vi "DisplacementSampleSensorLoop.vi"   [LabVIEW 2016]
uses:
  DisplacementSampleSensorLoopData.ctl
  DisplacementSampleSensorLoopStates.ctl
  DisplacementSample.ctl
  DisplacementErrorSample.ctl
  DisplacementErrorCodes.ctl
  <vilib>/Platform/TimedLoop/XDataNode/timing_clust.ctl
  <vilib>/Platform/TimedLoop/XDataNode/nitl_modes.ctl
  <vilib>/Platform/TimedLoop/XDataNode/wakeup.ctl
  <vilib>/rvi/Emulation/niFpgaSctlEmulationGetInTimedLoop.vi
  <vilib>/rvi/Emulation/niFpgaEmulationReportErrorSimple.vi
  <vilib>/rvi/Emulation/niFpgaGetClockAttributes.vi
  <vilib>/rvi/Emulation/niFpgaCriticalErrorInLSC.vi
  <vilib>/rvi/Emulation/niFpgaEmulationIsFPGAContextNoSignature.vi
  <vilib>/rvi/errors/niFpgaSetErrorForExecOnDevCompSimple.vi
  <vilib>/rvi/eio/common/nirviEmuReportErrorAndStop.vi
  <vilib>/rvi/DataTransferAndStorage/Container/Common/niFpgaContainerGetUniqueNameForEmu.vi
  <vilib>/rvi/FIFO/Fifo_Resource/nirvififoEmulationSetSize.vi
  <vilib>/rvi/FIFO/Fifo_Resource/nirviFifoEmulationQueueMgr.vi
  <instcachedir>/0/nirviFifoEmulationQueueMgr_E5CAEC123FF24DC58D834DCA3CDAA9B5.lvgen/nirviFifoEmulationQueueMgr_E5CAEC123FF24DC58D834DCA3CDAA9B5_004.vi
  <vilib>/Utility/error.llb/Clear Errors.vi
  <vilib>/rvi/FIFO/Fifo_Resource/nirvififoEmulationCreateLock.vi
  <vilib>/rvi/Emulation/niFpgaProcessEmulError.vi
  <vilib>/rvi/FIFO/Fifo_Resource/nirvififoEmulationObtainLock.vi
  <vilib>/rvi/FIFO/Fifo_Resource/nirvififoEmulationReleaseLock.vi
  <vilib>/rvi/occurrence/nirviWaitOnOccurrenceBase.vi
  <vilib>/rvi/errors/nirviReportUnexpectedCaseInternalError.vi
  <vilib>/rvi/errors/nirviReportUnexpectedCaseInternalError (U32).vi
  <vilib>/rvi/FIFO/Fifo_Resource/nirvififoEmulationDetermineInputValidOut.vi
  <instcachedir>/0/nirviFifoEmulationQueueMgr_E5CAEC123FF24DC58D834DCA3CDAA9B5.lvgen/nirviFifoEmulationQueueMgr_E5CAEC123FF24DC58D834DCA3CDAA9B5_009.vi
  <vilib>/rvi/Memory/Memory_Emulation/niFpgaMemoryEmulationCacheClearOnFirstRun.vi
  <vilib>/rvi/Memory/Memory_Emulation/nirvimemoryEmulationManagerCache_MakeExclusive.vi
  <vilib>/rvi/Memory/Memory_Emulation/niFpgaMemoryEmulationValidateCache.vi
  <vilib>/rvi/Memory/Memory_Emulation/nirvimemoryEmulationManagerCache_InsertValue.vi
  <vilib>/rvi/Memory/Memory_Emulation/nirvimemoryEmulationManagerCache_ReleaseExclusive.vi
  <vilib>/rvi/Memory/Memory_Emulation/nirvimemoryEmulationManagerCache_GetValue.vi
  <vilib>/rvi/Memory/Memory_Emulation/nirvimemoryEmulationManagerCache_SetValue.vi
  <vilib>/rvi/eio/common/nirviEmuTemplateMethod_errors.vi
  <instcachedir>/0/nirviFifoEmulationQueueMgr_E5CAEC123FF24DC58D834DCA3CDAA9B5.lvgen/nirviFifoEmulationQueueMgr_E5CAEC123FF24DC58D834DCA3CDAA9B5_028.vi
  <instcachedir>/0/nirviFifoEmulationQueueMgr_E5CAEC123FF24DC58D834DCA3CDAA9B5.lvgen/nirviFifoEmulationQueueMgr_E5CAEC123FF24DC58D834DCA3CDAA9B5_029.vi
  <vilib>/Platform/TimedLoop/XDataNode/XDataNode.xnode
  <vilib>/rvi/DataTransferAndStorage/Container/XNode/niFpgaContainer.xnode
  <vilib>/rvi/FIFO/Fifo_Resource/nirvififoEmulationRead.vi
  <vilib>/rvi/FIFO/Fifo_Resource/nirvififoEmulationWrite.vi
  <vilib>/rvi/DataTransferAndStorage/Register/Emulation/niFpgaRegisterEmulation.vi
  <vilib>/eio/EIONode/EIONode.xnode
  <vilib>/Platform/TimedLoop/XDataNode/XDNodeRunTimeDep.lvlib
types:
  T1 = typedef "DisplacementSampleSensorLoopData.ctl" = cluster{"State":T2, "Sensor":u8, "Negative":bool, "Timestamp":u64, "ErrorNumber":u8, "Timeout":i32, "Sample":T3, "ErrorSample":T4}
  T2 = typedef "DisplacementSampleSensorLoopStates.ctl" = enum16{"WaitForTrigger", "ClearRxFIFO", "WaitForClearComplete", "WriteM", "Write0", "WriteCR", "WriteNL", "ReadFirstCharacter", "ReadDataResponse", "ReadDeliminator", "ReadSign", "ReadHundreds", "ReadTens", "ReadOnes", "ReadDecimal", "ReadTenths", "ReadHundredths", "ReadThousandths", "ReadTenThousandths", "PrepareSample", "MoveSample", "ReadErrorR", "ReadErrorDeliminator1", "ReadErrorM", "ReadError0", "ReadErrorDeliminator2", "ReadErrorNumberTens", "ReadErrorNumberOnes", "ReadErrorCR", "ParseErrorNumber", "ResponseUnknownError", "ResponseInvalidError", "ResponseTimeoutError", "SensorIndicatesInvalidCommandError", "SensorIndicatesCommunicationTimeoutError", "SensorIndicatesDataLengthError", "SensorIndicatesNumberOfParametersError", "SensorIndicatesParameterError", "SensorIndicatesCommunicationError", "SensorIndicatesIDNumberError", "SensorIndicatesExpansionLineError", "SensorIndicatesWriteControlError", "PrepareErrorCode", "MoveErrorCode"}
  T3 = typedef "DisplacementSample.ctl" = cluster{"Timestamp":u64, "TxBytes":u64, "RxBytes":u64, "TxFrames":u64, "RxFrames":u64, "Sensor1Raw":i32, "Sensor2Raw":i32, "Sensor3Raw":i32, "Sensor4Raw":i32, "Sensor5Raw":i32, "Sensor6Raw":i32, "Sensor7Raw":i32, "Sensor8Raw":i32, "Sensor1Eng":sgl, "Sensor2Eng":sgl, "Sensor3Eng":sgl, "Sensor4Eng":sgl, "Sensor5Eng":sgl, "Sensor6Eng":sgl, "Sensor7Eng":sgl, "Sensor8Eng":sgl, "PositionX":sgl, "PositionY":sgl, "PositionZ":sgl, "RotationX":sgl, "RotationY":sgl, "RotationZ":sgl}
  T4 = typedef "DisplacementErrorSample.ctl" = cluster{"Timestamp":u64, "TxBytes":u64, "RxBytes":u64, "TxFrames":u64, "RxFrames":u64, "ErrorCode":T5}
  T5 = typedef "DisplacementErrorCodes.ctl" = enum16{"None", "ResponseUnknownError", "ResponseInvalidError", "ResponseTimeoutError", "SensorIndicatesInvalidCommandError", "SensorIndicatesCommunicationTimeoutError", "SensorIndicatesDataLengthError", "SensorIndicatesNumberOfParametersError", "SensorIndicatesParameterError", "SensorIndicatesCommunicationError", "SensorIndicatesIDNumberError", "SensorIndicatesExpansionLineError", "SensorIndicatesWriteControlError"}
  T6 = typedef "XDNodeRunTimeDep.lvlib/timing_clust.ctl" = cluster{"Expected End [f-1]":u64, "Actual End [f-1]":u64, "Finished Late? [f-1]":bool, "Expected End [i-1]":u64, "Actual End [i-1]":u64, "Finished Late? [i-1]":bool, "Expected Start [i]":u64, "Actual Start [i]":u64, "Expected Start [f]":u64, "Actual Start [f]":u64, "Source Name":string, "Structure Name":string, "Period":i64, "Deadline":i64, "Offset":i64, "Start":i64, "Priority":i32, "Timeout":i32, "Mode":T7, "Wakeup Reason":T8, "Error":errorcluster, "Source Type":string, "Secondary Source Type":string, "Global End Time":u64, "Global Start Time":u64, "Frame Duration":u64, "Iteration Duration":u64, "Assigned CPU":i32, "I/O Scan Engine Mode":u32}
  T7 = typedef "XDNodeRunTimeDep.lvlib/nitl_modes.ctl" = enum32{"No Change", "Process missed periods, maintain original phase", "Discard missed periods, maintain original phase", "Process missed periods, ignore original phase", "Discard missed periods, ignore original phase"}
  T8 = typedef "XDNodeRunTimeDep.lvlib/wakeup.ctl" = enum32{"Normal", "Aborted", "Asynchronous wakeup", "Timing source error", "Timed loop error", "Timeout"}
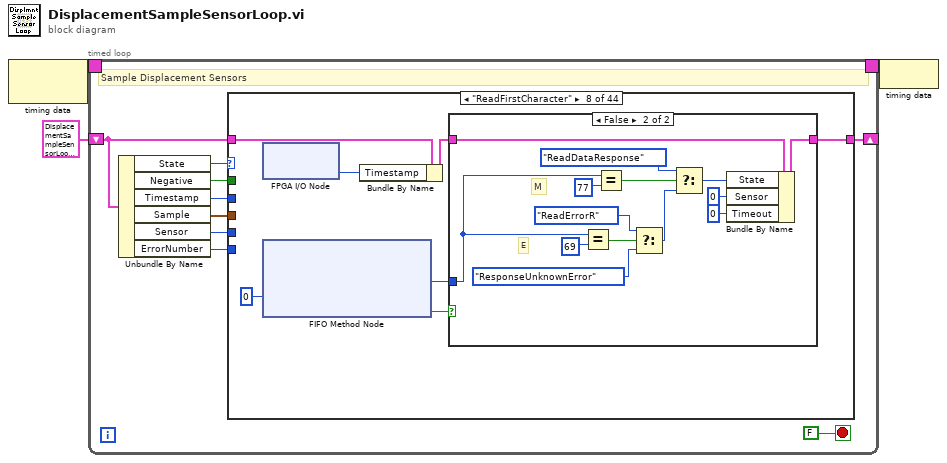
[diagram p0: block diagram]
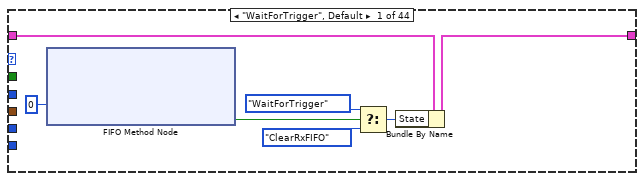
[diagram p2: hidden frame]
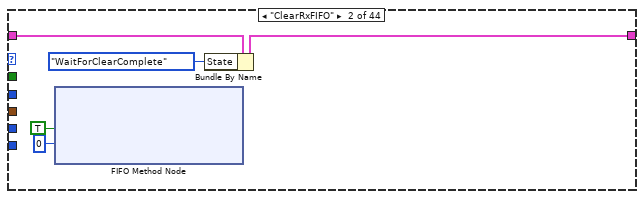
[diagram p3: hidden frame]
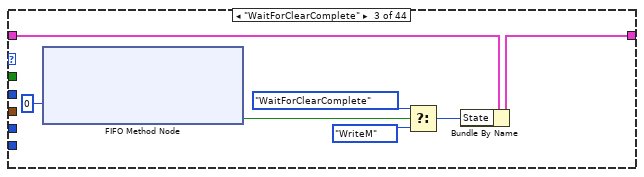
[diagram p4: hidden frame]
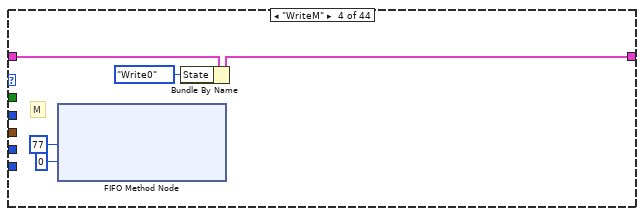
[diagram p5: hidden frame]
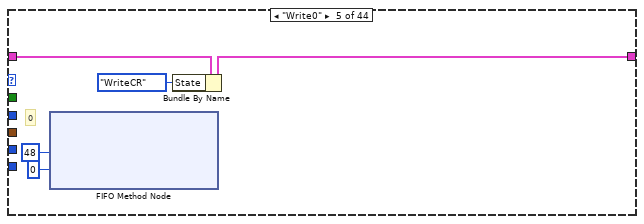
[diagram p6: hidden frame]
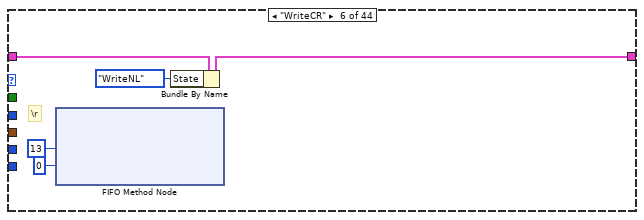
[diagram p7: hidden frame]
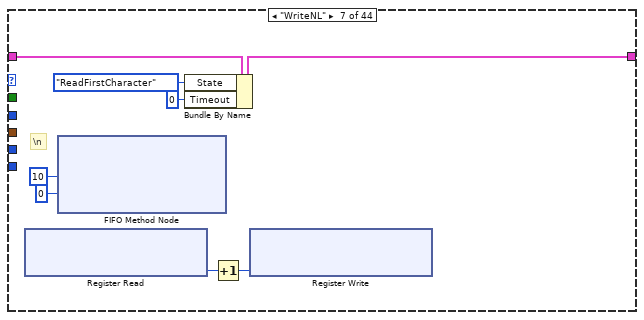
[diagram p8: hidden frame]
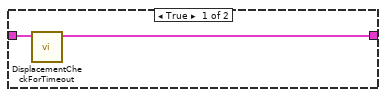
[diagram p9: hidden frame]
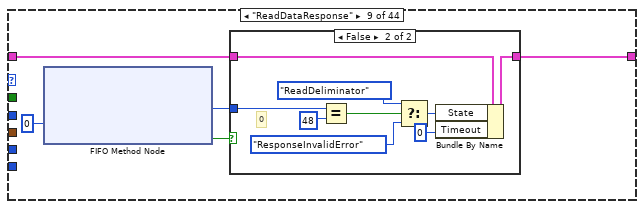
[diagram p10: hidden frame]
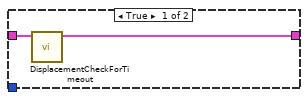
[diagram p11: hidden frame]
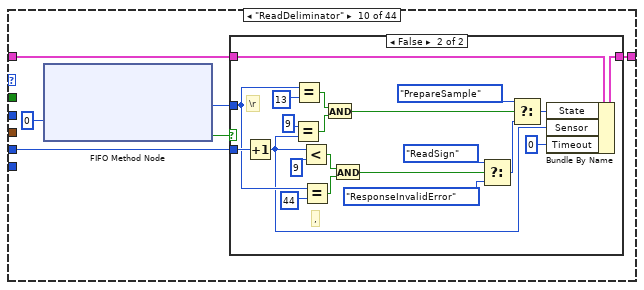
[diagram p12: hidden frame]
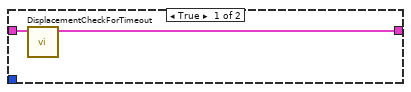
[diagram p13: hidden frame]
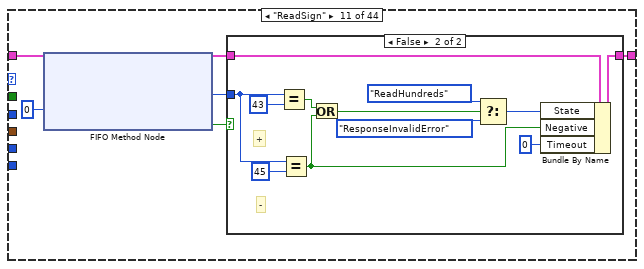
[diagram p14: hidden frame]
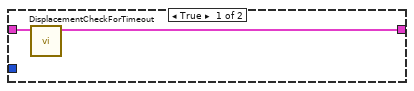
[diagram p15: hidden frame]
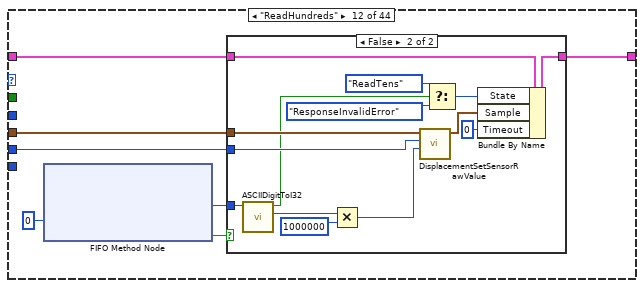
[diagram p16: hidden frame]
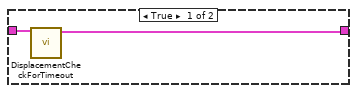
[diagram p17: hidden frame]
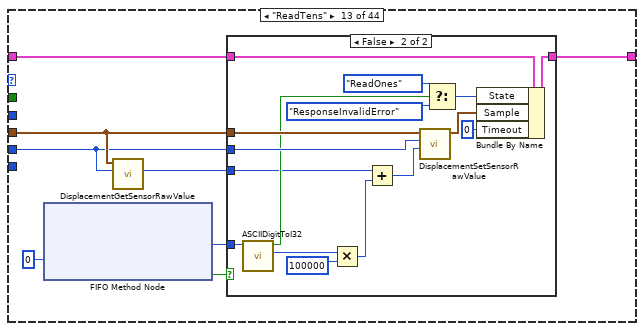
[diagram p18: hidden frame]
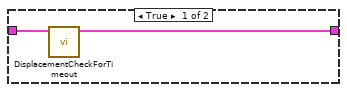
[diagram p19: hidden frame]
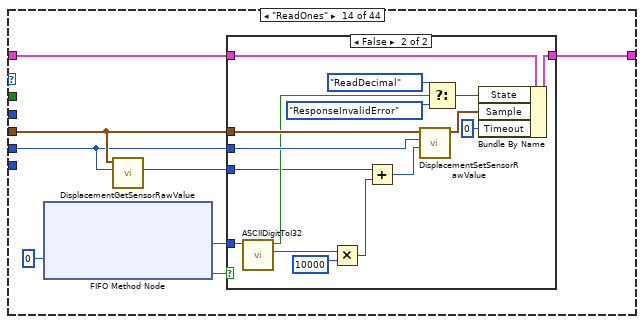
[diagram p20: hidden frame]
diagram:
  n1 = node-c288() -> (w3:T6)  [unwired: 1 in]
  n2 = timed-loop {
    timing: w3 -> [_]
    timing-out: [_] -> w2
    shift-right: [w12] -> _
    shift-left: T1 {"State"=enum."WaitForTrigger", "Sensor"=0, "Negative"=FALSE, "Timestamp"=0, "ErrorNumber"=0, "Timeout"=0, "Sample"={"Timestamp"=0, "TxBytes"=0, "RxBytes"=0, "TxFrames"=0, "RxFrames"=0, "Sensor1Raw"=0, "Sensor2Raw"=0, "Sensor3Raw"=0, "Sensor4Raw"=0, "Sensor5Raw"=0, "Sensor6Raw"=0, "Sensor7Raw"=0, "Sensor8Raw"=0, "Sensor1Eng"=0.0, "Sensor2Eng"=0.0, "Sensor3Eng"=0.0, "Sensor4Eng"=0.0, "Sensor5Eng"=0.0, "Sensor6Eng"=0.0, "Sensor7Eng"=0.0, "Sensor8Eng"=0.0, "PositionX"=0.0, "PositionY"=0.0, "PositionZ"=0.0, "RotationX"=0.0, "RotationY"=0.0, "RotationZ"=0.0}, "ErrorSample"={"Timestamp"=0, "TxBytes"=0, "RxBytes"=0, "TxFrames"=0, "RxFrames"=0, "ErrorCode"=enum."None"}} ("DisplacementData") -> [w11]
    stop <- FALSE stop-if-true
    # "Sample Displacement Sensors"
    n3 = Unbundle By Name(w11) -> ("State"=w10:T2, "Negative"=w9:bool, "Timestamp"=w7:u64, "Sample"=w8:T3, "Sensor"=w6:u8, "ErrorNumber"=w5:u8)
    n4 = case shown="\"ReadFirstCharacter\"" w10 {
      tunnel: [w16 w23 w30 w35 w40 w45 w53 w61 w81 w98 w126 w147 w171 w197 w220 w239 w265 w291 w317 w343 w350 w354 w370 w386 w402 w418 w434 w454 w473 w488 w502 w506 w510 w514 w518 w522 w526 w530 w534 w538 w542 w546 w556 w563] -> w12
      tunnel: w11 -> [w19 w24 w31 w36 w41 w46 w54 w57 w82 w99 w127 w148 w172 w198 w221 w240 w266 w292 w318 w344 w347 w355 w371 w387 w403 w419 w435 w455 w474 w489 w503 w507 w511 w515 w519 w523 w527 w531 w535 w539 w543 w547 w557 w560]
      tunnel: w9 -> [_ _ _ _ _ _ _ _ _ _ _ _ _ _ _ _ _ _ _ _ _ _ _ _ _ _ _ _ _ _ _ _ _ _ _ _ _ _ _ _ _ _ _ _]
      tunnel: w8 -> [_ _ _ _ _ _ _ _ _ _ _ w143 w167 w193 _ w235 w261 w287 w313 _ _ _ _ _ _ _ _ _ _ _ _ _ _ _ _ _ _ _ _ _ _ _ _ _]
      tunnel: w7 -> [_ _ _ _ _ _ _ _ _ _ _ _ _ _ _ _ _ _ _ w335 _ _ _ _ _ _ _ _ _ _ _ _ _ _ _ _ _ _ _ _ _ _ w548 _]
      tunnel: w6 -> [_ _ _ _ _ _ _ _ _ w94 _ w142 w166 w192 _ w234 w260 w286 w312 _ _ _ _ _ _ _ _ _ _ _ _ _ _ _ _ _ _ _ _ _ _ _ _ _]
      tunnel: w5 -> [_ _ _ _ _ _ _ _ _ _ _ _ _ _ _ _ _ _ _ _ _ _ _ _ _ _ _ w450 _ w486 _ _ _ _ _ _ _ _ _ _ _ _ _ _]
      frame "WaitForTrigger", Default {
        n5 = xnode ("FIFO Method Node")("Timeout"=0) -> ("Timed Out?"=w14:bool)  [unwired: 1 in, 2 out]
        n6 = Select(t=DisplacementSampleSensorLoopStates."WaitForTrigger" ("DisplacementStates"), s=w14, f=DisplacementSampleSensorLoopStates."ClearRxFIFO") -> (s? t:f=w17:T2)
        n7 = Bundle By Name(cluster=w19, "State"=w17) -> (w16:T1)
      }
      frame "ClearRxFIFO" {
        n8 = xnode ("FIFO Method Node")("Element"=TRUE, "Timeout"=0) -> ()  [unwired: 1 in, 2 out]
        n9 = Bundle By Name(cluster=w24, "State"=DisplacementSampleSensorLoopStates."WaitForClearComplete") -> (w23:T1)
      }
      frame "WaitForClearComplete" {
        n10 = xnode ("FIFO Method Node")("Timeout"=0) -> ("Timed Out?"=w26:bool)  [unwired: 1 in, 2 out]
        n11 = Select(t=DisplacementSampleSensorLoopStates."WaitForClearComplete" ("State"), s=w26, f=DisplacementSampleSensorLoopStates."WriteM") -> (s? t:f=w28:T2)
        n12 = Bundle By Name(cluster=w31, "State"=w28) -> (w30:T1)
      }
      frame "WriteM" {
        # "M"
        n13 = xnode ("FIFO Method Node")("Element"=u8 77, "Timeout"=0) -> ()  [unwired: 1 in, 2 out]
        n14 = Bundle By Name(cluster=w36, "State"=DisplacementSampleSensorLoopStates."Write0" ("f")) -> (w35:T1)
      }
      frame "Write0" {
        # "0"
        n15 = xnode ("FIFO Method Node")("Element"=u8 48, "Timeout"=0) -> ()  [unwired: 1 in, 2 out]
        n16 = Bundle By Name(cluster=w41, "State"=DisplacementSampleSensorLoopStates."WriteCR" ("f")) -> (w40:T1)
      }
      frame "WriteCR" {
        # "\\r"
        n17 = xnode ("FIFO Method Node")("Element"=u8 13, "Timeout"=0) -> ()  [unwired: 1 in, 2 out]
        n18 = Bundle By Name(cluster=w46, "State"=DisplacementSampleSensorLoopStates."WriteNL" ("f")) -> (w45:T1)
      }
      frame "WriteNL" {
        # "\\n"
        n19 = xnode ("Register Read")() -> ("Data"=w48:u64)  [unwired: 1 in, 1 out]
        n20 = xnode ("FIFO Method Node")("Element"=u8 10, "Timeout"=0) -> ()  [unwired: 1 in, 2 out]
        n21 = Bundle By Name(cluster=w54, "State"=DisplacementSampleSensorLoopStates."ReadFirstCharacter", "Timeout"=0) -> (w53:T1)
        n22 = Increment(x=w48) -> (x+1=w49:u64)
        n23 = xnode ("Register Write")("Data"=w49) -> ()  [unwired: 1 in, 1 out]
      }
      frame "ReadFirstCharacter" {
        n24 = xnode "FPGA I/O Node"() -> ("Time"=w55:u64)  [unwired: 1 in, 1 out]
        n25 = xnode ("FIFO Method Node")("Timeout"=0) -> ("Element"=w58:u8, "Timed Out?"=w59:bool)  [unwired: 1 in, 1 out]
        n26 = Bundle By Name(cluster=w57, "Timestamp"=w55) -> (w56:T1)
        n27 = case shown="False" w59 {
          tunnel: w56 -> [w63 w64]
          tunnel: [w62 w77] -> w61
          tunnel: w58 -> [_ w70]
          frame True {
            n28 = call "DisplacementCheckForTimeout.vi"("DisplacementSampleSensorLoopData in"=w63) -> ("DisplacementSampleSensorLoopData out"=w62:T1)  [unwired: 10 in]
          }
          frame False {
            # "E"
            # "M"
            n29 = Equal?(x=w70, y=u8 69) -> (x = y?=w71:bool)
            n30 = Equal?(x=w70, y=u8 77) -> (x = y?=w75:bool)
            n31 = Select(t=DisplacementSampleSensorLoopStates."ReadErrorR", s=w71, f=DisplacementSampleSensorLoopStates."ResponseUnknownError") -> (s? t:f=w68:T2)
            n32 = Select(t=DisplacementSampleSensorLoopStates."ReadDataResponse" ("State"), s=w75, f=w68) -> (s? t:f=w74:T2)
            n33 = Bundle By Name(cluster=w64, "State"=w74, "Sensor"=u8 0, "Timeout"=0) -> (w77:T1)
          }
        }
      }
      frame "ReadDataResponse" {
        n34 = xnode ("FIFO Method Node")("Timeout"=0) -> ("Element"=w78:u8, "Timed Out?"=w79:bool)  [unwired: 1 in, 1 out]
        n35 = case shown="False" w79 {
          tunnel: w82 -> [w84 w93]
          tunnel: [w83 w92] -> w81
          tunnel: w78 -> [_ w87]
          frame True {
            n36 = call "DisplacementCheckForTimeout.vi"("DisplacementSampleSensorLoopData in"=w84) -> ("DisplacementSampleSensorLoopData out"=w83:T1)  [unwired: 10 in]
          }
          frame False {
            # "0"
            n37 = Equal?(x=w87, y=u8 48) -> (x = y?=w90:bool)
            n38 = Select(t=DisplacementSampleSensorLoopStates."ReadDeliminator" ("State"), s=w90, f=DisplacementSampleSensorLoopStates."ResponseInvalidError") -> (s? t:f=w89:T2)
            n39 = Bundle By Name(cluster=w93, "State"=w89, "Timeout"=0) -> (w92:T1)
          }
        }
      }
      frame "ReadDeliminator" {
        n40 = xnode ("FIFO Method Node")("Timeout"=0) -> ("Element"=w95:u8, "Timed Out?"=w96:bool)  [unwired: 1 in, 1 out]
        n41 = case shown="False" w96 {
          tunnel: w99 -> [w101 w122]
          tunnel: [w100 w121] -> w98
          tunnel: w95 -> [_ w111]
          tunnel: w94 -> [_ w118]
          frame True {
            n42 = call "DisplacementCheckForTimeout.vi"("DisplacementSampleSensorLoopData in"=w101) -> ("DisplacementSampleSensorLoopData out"=w100:T1)  [unwired: 10 in]
          }
          frame False {
            # "\\r"
            # ","
            n43 = Increment(x=w118) -> (x+1=w103:u8)
            n44 = Equal?(x=u8 9, y=w103) -> (x = y?=w110:bool)
            n45 = Equal?(x=w111, y=u8 13) -> (x = y?=w109:bool)
            n46 = Less?(x=w103, y=u8 9) -> (x < y?=w116:bool)
            n47 = Equal?(x=w111, y=u8 44) -> (x = y?=w115:bool)
            n48 = And(x=w109, y=w110) -> (x .and. y?=w107:bool)
            n49 = And(x=w116, y=w115) -> (x .and. y?=w104:bool)
            n50 = Select(t=DisplacementSampleSensorLoopStates."ReadSign" ("State"), s=w104, f=DisplacementSampleSensorLoopStates."ResponseInvalidError") -> (s? t:f=w108:T2)
            n51 = Select(t=DisplacementSampleSensorLoopStates."PrepareSample", s=w107, f=w108) -> (s? t:f=w105:T2)
            n52 = Bundle By Name(cluster=w122, "State"=w105, "Sensor"=w103, "Timeout"=0) -> (w121:T1)
          }
        }
      }
      frame "ReadSign" {
        n53 = xnode ("FIFO Method Node")("Timeout"=0) -> ("Element"=w123:u8, "Timed Out?"=w124:bool)  [unwired: 1 in, 1 out]
        n54 = case shown="False" w124 {
          tunnel: w127 -> [w129 w141]
          tunnel: [w128 w140] -> w126
          tunnel: w123 -> [_ w137]
          frame True {
            n55 = call "DisplacementCheckForTimeout.vi"("DisplacementSampleSensorLoopData in"=w129) -> ("DisplacementSampleSensorLoopData out"=w128:T1)  [unwired: 10 in]
          }
          frame False {
            # "+"
            # "-"
            n56 = Equal?(x=w137, y=u8 43) -> (x = y?=w138:bool)
            n57 = Equal?(x=w137, y=u8 45) -> (x = y?=w135:bool)
            n58 = Or(x=w138, y=w135) -> (x .or. y?=w134:bool)
            n59 = Select(t=DisplacementSampleSensorLoopStates."ReadHundreds" ("State"), s=w134, f=DisplacementSampleSensorLoopStates."ResponseInvalidError") -> (s? t:f=w132:T2)
            n60 = Bundle By Name(cluster=w141, "State"=w132, "Negative"=w135, "Timeout"=0) -> (w140:T1)
          }
        }
      }
      frame "ReadHundreds" {
        n61 = xnode ("FIFO Method Node")("Timeout"=0) -> ("Element"=w144:u8, "Timed Out?"=w145:bool)  [unwired: 1 in, 1 out]
        n62 = case shown="False" w145 {
          tunnel: w148 -> [w150 w164]
          tunnel: [w149 w163] -> w147
          tunnel: w144 -> [_ w154]
          tunnel: w143 -> [_ w157]
          tunnel: w142 -> [_ w155]
          frame True {
            n63 = call "DisplacementCheckForTimeout.vi"("DisplacementSampleSensorLoopData in"=w150) -> ("DisplacementSampleSensorLoopData out"=w149:T1)  [unwired: 10 in]
          }
          frame False {
            n64 = call "ASCIIDigitToI32.vi"("Value"=w154) -> ("Number"=w152:i32, "Valid"=w153:bool)  [unwired: 9 in]
            n65 = Multiply(x=w152, y=1000000) -> (x*y=w158:i32)
            n66 = call "DisplacementSetSensorRawValue.vi"("Value"=w158, "Sensor"=w155, "DisplacementSample in"=w157) -> ("DisplacementSample out"=w156:T3)  [unwired: 8 in]
            n67 = Select(t=DisplacementSampleSensorLoopStates."ReadTens" ("State"), s=w153, f=DisplacementSampleSensorLoopStates."ResponseInvalidError" ("State")) -> (s? t:f=w161:T2)
            n68 = Bundle By Name(cluster=w164, "State"=w161, "Sample"=w156, "Timeout"=0) -> (w163:T1)
          }
        }
      }
      frame "ReadTens" {
        n69 = xnode ("FIFO Method Node")("Timeout"=0) -> ("Element"=w168:u8, "Timed Out?"=w169:bool)  [unwired: 1 in, 1 out]
        n70 = call "DisplacementGetSensorRawValue.vi"("Sensor"=w166, "DisplacementSample"=w167) -> ("Value"=w165:i32)  [unwired: 9 in]
        n71 = case shown="False" w169 {
          tunnel: w172 -> [w174 w190]
          tunnel: [w173 w189] -> w171
          tunnel: w168 -> [_ w181]
          tunnel: w167 -> [_ w184]
          tunnel: w166 -> [_ w182]
          tunnel: w165 -> [_ w178]
          frame True {
            n72 = call "DisplacementCheckForTimeout.vi"("DisplacementSampleSensorLoopData in"=w174) -> ("DisplacementSampleSensorLoopData out"=w173:T1)  [unwired: 10 in]
          }
          frame False {
            n73 = call "ASCIIDigitToI32.vi"("Value"=w181) -> ("Number"=w179:i32, "Valid"=w180:bool)  [unwired: 9 in]
            n74 = Multiply(x=w179, y=100000) -> (x*y=w176:i32)
            n75 = Add(x=w178, y=w176) -> (x+y=w177:i32)
            n76 = call "DisplacementSetSensorRawValue.vi"("Value"=w177, "Sensor"=w182, "DisplacementSample in"=w184) -> ("DisplacementSample out"=w183:T3)  [unwired: 8 in]
            n77 = Select(t=DisplacementSampleSensorLoopStates."ReadOnes" ("State"), s=w180, f=DisplacementSampleSensorLoopStates."ResponseInvalidError" ("State")) -> (s? t:f=w187:T2)
            n78 = Bundle By Name(cluster=w190, "State"=w187, "Sample"=w183, "Timeout"=0) -> (w189:T1)
          }
        }
      }
      frame "ReadOnes" {
        n79 = xnode ("FIFO Method Node")("Timeout"=0) -> ("Element"=w194:u8, "Timed Out?"=w195:bool)  [unwired: 1 in, 1 out]
        n80 = call "DisplacementGetSensorRawValue.vi"("Sensor"=w192, "DisplacementSample"=w193) -> ("Value"=w191:i32)  [unwired: 9 in]
        n81 = case shown="False" w195 {
          tunnel: w198 -> [w200 w216]
          tunnel: [w199 w215] -> w197
          tunnel: w194 -> [_ w207]
          tunnel: w193 -> [_ w210]
          tunnel: w192 -> [_ w208]
          tunnel: w191 -> [_ w204]
          frame True {
            n82 = call "DisplacementCheckForTimeout.vi"("DisplacementSampleSensorLoopData in"=w200) -> ("DisplacementSampleSensorLoopData out"=w199:T1)  [unwired: 10 in]
          }
          frame False {
            n83 = call "ASCIIDigitToI32.vi"("Value"=w207) -> ("Number"=w205:i32, "Valid"=w206:bool)  [unwired: 9 in]
            n84 = Multiply(x=w205, y=10000) -> (x*y=w202:i32)
            n85 = Add(x=w204, y=w202) -> (x+y=w203:i32)
            n86 = call "DisplacementSetSensorRawValue.vi"("Value"=w203, "Sensor"=w208, "DisplacementSample in"=w210) -> ("DisplacementSample out"=w209:T3)  [unwired: 8 in]
            n87 = Select(t=DisplacementSampleSensorLoopStates."ReadDecimal" ("State"), s=w206, f=DisplacementSampleSensorLoopStates."ResponseInvalidError" ("State")) -> (s? t:f=w213:T2)
            n88 = Bundle By Name(cluster=w216, "State"=w213, "Sample"=w209, "Timeout"=0) -> (w215:T1)
          }
        }
      }
      frame "ReadDecimal" {
        n89 = xnode ("FIFO Method Node")("Timeout"=0) -> ("Element"=w217:u8, "Timed Out?"=w218:bool)  [unwired: 1 in, 1 out]
        n90 = case shown="False" w218 {
          tunnel: w221 -> [w223 w232]
          tunnel: [w222 w231] -> w220
          tunnel: w217 -> [_ w227]
          frame True {
            n91 = call "DisplacementCheckForTimeout.vi"("DisplacementSampleSensorLoopData in"=w223) -> ("DisplacementSampleSensorLoopData out"=w222:T1)  [unwired: 10 in]
          }
          frame False {
            # "."
            n92 = Equal?(x=w227, y=u8 46) -> (x = y?=w225:bool)
            n93 = Select(t=DisplacementSampleSensorLoopStates."ReadTenths" ("State"), s=w225, f=DisplacementSampleSensorLoopStates."ResponseInvalidError" ("State")) -> (s? t:f=w230:T2)
            n94 = Bundle By Name(cluster=w232, "State"=w230, "Timeout"=0) -> (w231:T1)
          }
        }
      }
      frame "ReadTenths" {
        n95 = xnode ("FIFO Method Node")("Timeout"=0) -> ("Element"=w236:u8, "Timed Out?"=w237:bool)  [unwired: 1 in, 1 out]
        n96 = call "DisplacementGetSensorRawValue.vi"("Sensor"=w234, "DisplacementSample"=w235) -> ("Value"=w233:i32)  [unwired: 9 in]
        n97 = case shown="False" w237 {
          tunnel: w240 -> [w242 w258]
          tunnel: [w241 w257] -> w239
          tunnel: w236 -> [_ w249]
          tunnel: w235 -> [_ w252]
          tunnel: w234 -> [_ w250]
          tunnel: w233 -> [_ w246]
          frame True {
            n98 = call "DisplacementCheckForTimeout.vi"("DisplacementSampleSensorLoopData in"=w242) -> ("DisplacementSampleSensorLoopData out"=w241:T1)  [unwired: 10 in]
          }
          frame False {
            n99 = call "ASCIIDigitToI32.vi"("Value"=w249) -> ("Number"=w247:i32, "Valid"=w248:bool)  [unwired: 9 in]
            n100 = Multiply(x=w247, y=1000) -> (x*y=w244:i32)
            n101 = Add(x=w246, y=w244) -> (x+y=w245:i32)
            n102 = call "DisplacementSetSensorRawValue.vi"("Value"=w245, "Sensor"=w250, "DisplacementSample in"=w252) -> ("DisplacementSample out"=w251:T3)  [unwired: 8 in]
            n103 = Select(t=DisplacementSampleSensorLoopStates."ReadHundredths" ("State"), s=w248, f=DisplacementSampleSensorLoopStates."ResponseInvalidError" ("State")) -> (s? t:f=w255:T2)
            n104 = Bundle By Name(cluster=w258, "State"=w255, "Sample"=w251, "Timeout"=0) -> (w257:T1)
          }
        }
      }
      frame "ReadHundredths" {
        n105 = xnode ("FIFO Method Node")("Timeout"=0) -> ("Element"=w262:u8, "Timed Out?"=w263:bool)  [unwired: 1 in, 1 out]
        n106 = call "DisplacementGetSensorRawValue.vi"("Sensor"=w260, "DisplacementSample"=w261) -> ("Value"=w259:i32)  [unwired: 9 in]
        n107 = case shown="False" w263 {
          tunnel: w266 -> [w268 w284]
          tunnel: [w267 w283] -> w265
          tunnel: w262 -> [_ w275]
          tunnel: w261 -> [_ w278]
          tunnel: w260 -> [_ w276]
          tunnel: w259 -> [_ w272]
          frame True {
            n108 = call "DisplacementCheckForTimeout.vi"("DisplacementSampleSensorLoopData in"=w268) -> ("DisplacementSampleSensorLoopData out"=w267:T1)  [unwired: 10 in]
          }
          frame False {
            n109 = call "ASCIIDigitToI32.vi"("Value"=w275) -> ("Number"=w273:i32, "Valid"=w274:bool)  [unwired: 9 in]
            n110 = Multiply(x=w273, y=100) -> (x*y=w270:i32)
            n111 = Add(x=w272, y=w270) -> (x+y=w271:i32)
            n112 = call "DisplacementSetSensorRawValue.vi"("Value"=w271, "Sensor"=w276, "DisplacementSample in"=w278) -> ("DisplacementSample out"=w277:T3)  [unwired: 8 in]
            n113 = Select(t=DisplacementSampleSensorLoopStates."ReadThousandths" ("State"), s=w274, f=DisplacementSampleSensorLoopStates."ResponseInvalidError" ("State")) -> (s? t:f=w281:T2)
            n114 = Bundle By Name(cluster=w284, "State"=w281, "Sample"=w277, "Timeout"=0) -> (w283:T1)
          }
        }
      }
      frame "ReadThousandths" {
        n115 = xnode ("FIFO Method Node")("Timeout"=0) -> ("Element"=w288:u8, "Timed Out?"=w289:bool)  [unwired: 1 in, 1 out]
        n116 = call "DisplacementGetSensorRawValue.vi"("Sensor"=w286, "DisplacementSample"=w287) -> ("Value"=w285:i32)  [unwired: 9 in]
        n117 = case shown="False" w289 {
          tunnel: w292 -> [w294 w310]
          tunnel: [w293 w309] -> w291
          tunnel: w288 -> [_ w301]
          tunnel: w287 -> [_ w304]
          tunnel: w286 -> [_ w302]
          tunnel: w285 -> [_ w298]
          frame True {
            n118 = call "DisplacementCheckForTimeout.vi"("DisplacementSampleSensorLoopData in"=w294) -> ("DisplacementSampleSensorLoopData out"=w293:T1)  [unwired: 10 in]
          }
          frame False {
            n119 = call "ASCIIDigitToI32.vi"("Value"=w301) -> ("Number"=w299:i32, "Valid"=w300:bool)  [unwired: 9 in]
            n120 = Multiply(x=w299, y=10) -> (x*y=w296:i32)
            n121 = Add(x=w298, y=w296) -> (x+y=w297:i32)
            n122 = call "DisplacementSetSensorRawValue.vi"("Value"=w297, "Sensor"=w302, "DisplacementSample in"=w304) -> ("DisplacementSample out"=w303:T3)  [unwired: 8 in]
            n123 = Select(t=DisplacementSampleSensorLoopStates."ReadTenThousandths" ("State"), s=w300, f=DisplacementSampleSensorLoopStates."ResponseInvalidError" ("State")) -> (s? t:f=w307:T2)
            n124 = Bundle By Name(cluster=w310, "State"=w307, "Sample"=w303, "Timeout"=0) -> (w309:T1)
          }
        }
      }
      frame "ReadTenThousandths" {
        n125 = xnode ("FIFO Method Node")("Timeout"=0) -> ("Element"=w314:u8, "Timed Out?"=w315:bool)  [unwired: 1 in, 1 out]
        n126 = call "DisplacementGetSensorRawValue.vi"("Sensor"=w312, "DisplacementSample"=w313) -> ("Value"=w311:i32)  [unwired: 9 in]
        n127 = case shown="False" w315 {
          tunnel: w318 -> [w320 w334]
          tunnel: [w319 w333] -> w317
          tunnel: w314 -> [_ w326]
          tunnel: w313 -> [_ w329]
          tunnel: w312 -> [_ w327]
          tunnel: w311 -> [_ w324]
          frame True {
            n128 = call "DisplacementCheckForTimeout.vi"("DisplacementSampleSensorLoopData in"=w320) -> ("DisplacementSampleSensorLoopData out"=w319:T1)  [unwired: 10 in]
          }
          frame False {
            n129 = call "ASCIIDigitToI32.vi"("Value"=w326) -> ("Number"=w322:i32, "Valid"=w325:bool)  [unwired: 9 in]
            n130 = Add(x=w324, y=w322) -> (x+y=w323:i32)
            n131 = call "DisplacementSetSensorRawValue.vi"("Value"=w323, "Sensor"=w327, "DisplacementSample in"=w329) -> ("DisplacementSample out"=w328:T3)  [unwired: 8 in]
            n132 = Select(t=DisplacementSampleSensorLoopStates."ReadDeliminator" ("State"), s=w325, f=DisplacementSampleSensorLoopStates."ResponseInvalidError" ("State")) -> (s? t:f=w332:T2)
            n133 = Bundle By Name(cluster=w334, "State"=w332, "Sample"=w328, "Timeout"=0) -> (w333:T1)
          }
        }
      }
      frame "PrepareSample" {
        n134 = xnode ("Register Read")() -> ("Data"=w341:u64)  [unwired: 1 in, 1 out]
        n135 = xnode ("Register Read")() -> ("Data"=w337:u64)  [unwired: 1 in, 1 out]
        n136 = xnode ("Register Read")() -> ("Data"=w338:u64)  [unwired: 1 in, 1 out]
        n137 = xnode ("Register Read")() -> ("Data"=w336:u64)  [unwired: 1 in, 1 out]
        n138 = Increment(x=w341) -> (x+1=w339:u64)
        n139 = xnode ("Register Write")("Data"=w339) -> ()  [unwired: 1 in, 1 out]
        n140 = Bundle By Name(cluster=w344, "State"=DisplacementSampleSensorLoopStates."MoveSample", "Sensor"=u8 1, "Sample.RxFrames"=w339, "Sample.TxBytes"=w338, "Sample.RxBytes"=w337, "Sample.TxFrames"=w336, "Sample.Timestamp"=w335) -> (w343:T1)
      }
      frame "MoveSample" {
        n141 = Unbundle By Name(w347) -> ("Sample"=w345:T3)
        n142 = xnode ("FIFO Method Node")("Element"=w345, "Timeout"=0) -> ()  [unwired: 1 in, 2 out]
        n143 = Bundle By Name(cluster=w347, "State"=DisplacementSampleSensorLoopStates."WaitForTrigger", "Sensor"=u8 1) -> (w350:T1)
      }
      frame "ReadErrorR" {
        n144 = xnode ("FIFO Method Node")("Timeout"=0) -> ("Element"=w351:u8, "Timed Out?"=w352:bool)  [unwired: 1 in, 1 out]
        n145 = case shown="False" w352 {
          tunnel: w355 -> [w357 w366]
          tunnel: [w356 w365] -> w354
          tunnel: w351 -> [_ w360]
          frame True {
            n146 = call "DisplacementCheckForTimeout.vi"("DisplacementSampleSensorLoopData in"=w357) -> ("DisplacementSampleSensorLoopData out"=w356:T1)  [unwired: 10 in]
          }
          frame False {
            # "R"
            n147 = Equal?(x=w360, y=u8 82) -> (x = y?=w363:bool)
            n148 = Select(t=DisplacementSampleSensorLoopStates."ReadErrorDeliminator1" ("State"), s=w363, f=DisplacementSampleSensorLoopStates."ResponseInvalidError") -> (s? t:f=w362:T2)
            n149 = Bundle By Name(cluster=w366, "State"=w362, "Timeout"=0) -> (w365:T1)
          }
        }
      }
      frame "ReadErrorDeliminator1" {
        n150 = xnode ("FIFO Method Node")("Timeout"=0) -> ("Element"=w367:u8, "Timed Out?"=w368:bool)  [unwired: 1 in, 1 out]
        n151 = case shown="False" w368 {
          tunnel: w371 -> [w373 w382]
          tunnel: [w372 w381] -> w370
          tunnel: w367 -> [_ w377]
          frame True {
            n152 = call "DisplacementCheckForTimeout.vi"("DisplacementSampleSensorLoopData in"=w373) -> ("DisplacementSampleSensorLoopData out"=w372:T1)  [unwired: 10 in]
          }
          frame False {
            # ","
            n153 = Equal?(x=w377, y=u8 44) -> (x = y?=w376:bool)
            n154 = Select(t=DisplacementSampleSensorLoopStates."ReadErrorM" ("State"), s=w376, f=DisplacementSampleSensorLoopStates."ResponseInvalidError") -> (s? t:f=w375:T2)
            n155 = Bundle By Name(cluster=w382, "State"=w375, "Timeout"=0) -> (w381:T1)
          }
        }
      }
      frame "ReadErrorM" {
        n156 = xnode ("FIFO Method Node")("Timeout"=0) -> ("Element"=w383:u8, "Timed Out?"=w384:bool)  [unwired: 1 in, 1 out]
        n157 = case shown="False" w384 {
          tunnel: w387 -> [w389 w398]
          tunnel: [w388 w397] -> w386
          tunnel: w383 -> [_ w392]
          frame True {
            n158 = call "DisplacementCheckForTimeout.vi"("DisplacementSampleSensorLoopData in"=w389) -> ("DisplacementSampleSensorLoopData out"=w388:T1)  [unwired: 10 in]
          }
          frame False {
            # "M"
            n159 = Equal?(x=w392, y=u8 77) -> (x = y?=w395:bool)
            n160 = Select(t=DisplacementSampleSensorLoopStates."ReadError0" ("State"), s=w395, f=DisplacementSampleSensorLoopStates."ResponseInvalidError") -> (s? t:f=w394:T2)
            n161 = Bundle By Name(cluster=w398, "State"=w394, "Timeout"=0) -> (w397:T1)
          }
        }
      }
      frame "ReadError0" {
        n162 = xnode ("FIFO Method Node")("Timeout"=0) -> ("Element"=w399:u8, "Timed Out?"=w400:bool)  [unwired: 1 in, 1 out]
        n163 = case shown="False" w400 {
          tunnel: w403 -> [w405 w414]
          tunnel: [w404 w413] -> w402
          tunnel: w399 -> [_ w408]
          frame True {
            n164 = call "DisplacementCheckForTimeout.vi"("DisplacementSampleSensorLoopData in"=w405) -> ("DisplacementSampleSensorLoopData out"=w404:T1)  [unwired: 10 in]
          }
          frame False {
            # "0"
            n165 = Equal?(x=w408, y=u8 48) -> (x = y?=w411:bool)
            n166 = Select(t=DisplacementSampleSensorLoopStates."ReadErrorDeliminator2" ("State"), s=w411, f=DisplacementSampleSensorLoopStates."ResponseInvalidError") -> (s? t:f=w410:T2)
            n167 = Bundle By Name(cluster=w414, "State"=w410, "Timeout"=0) -> (w413:T1)
          }
        }
      }
      frame "ReadErrorDeliminator2" {
        n168 = xnode ("FIFO Method Node")("Timeout"=0) -> ("Element"=w415:u8, "Timed Out?"=w416:bool)  [unwired: 1 in, 1 out]
        n169 = case shown="False" w416 {
          tunnel: w419 -> [w421 w430]
          tunnel: [w420 w429] -> w418
          tunnel: w415 -> [_ w425]
          frame True {
            n170 = call "DisplacementCheckForTimeout.vi"("DisplacementSampleSensorLoopData in"=w421) -> ("DisplacementSampleSensorLoopData out"=w420:T1)  [unwired: 10 in]
          }
          frame False {
            # ","
            n171 = Equal?(x=w425, y=u8 44) -> (x = y?=w424:bool)
            n172 = Select(t=DisplacementSampleSensorLoopStates."ReadErrorNumberTens" ("State"), s=w424, f=DisplacementSampleSensorLoopStates."ResponseInvalidError") -> (s? t:f=w423:T2)
            n173 = Bundle By Name(cluster=w430, "State"=w423, "Timeout"=0) -> (w429:T1)
          }
        }
      }
      frame "ReadErrorNumberTens" {
        n174 = xnode ("FIFO Method Node")("Timeout"=0) -> ("Element"=w431:u8, "Timed Out?"=w432:bool)  [unwired: 1 in, 1 out]
        n175 = case shown="False" w432 {
          tunnel: w435 -> [w437 w449]
          tunnel: [w436 w448] -> w434
          tunnel: w431 -> [_ w442]
          frame True {
            n176 = call "DisplacementCheckForTimeout.vi"("DisplacementSampleSensorLoopData in"=w437) -> ("DisplacementSampleSensorLoopData out"=w436:T1)  [unwired: 10 in]
          }
          frame False {
            n177 = call "ASCIIDigitToI32.vi"("Value"=w442) -> ("Number"=w439:i32, "Valid"=w441:bool)  [unwired: 9 in]
            n178 = To Unsigned Byte Integer(number=w439) -> (unsigned 8bit integer=w440:u8)
            n179 = Multiply(x=w440, y=u8 10) -> (x*y=w443:u8)
            n180 = Select(t=DisplacementSampleSensorLoopStates."ReadErrorNumberOnes" ("State"), s=w441, f=DisplacementSampleSensorLoopStates."ResponseInvalidError" ("State")) -> (s? t:f=w446:T2)
            n181 = Bundle By Name(cluster=w449, "State"=w446, "ErrorNumber"=w443, "Timeout"=0) -> (w448:T1)
          }
        }
      }
      frame "ReadErrorNumberOnes" {
        n182 = xnode ("FIFO Method Node")("Timeout"=0) -> ("Element"=w451:u8, "Timed Out?"=w452:bool)  [unwired: 1 in, 1 out]
        n183 = case shown="False" w452 {
          tunnel: w455 -> [w457 w469]
          tunnel: [w456 w468] -> w454
          tunnel: w451 -> [_ w462]
          tunnel: w450 -> [_ w463]
          frame True {
            n184 = call "DisplacementCheckForTimeout.vi"("DisplacementSampleSensorLoopData in"=w457) -> ("DisplacementSampleSensorLoopData out"=w456:T1)  [unwired: 10 in]
          }
          frame False {
            n185 = call "ASCIIDigitToI32.vi"("Value"=w462) -> ("Number"=w460:i32, "Valid"=w461:bool)  [unwired: 9 in]
            n186 = To Unsigned Byte Integer(number=w460) -> (unsigned 8bit integer=w459:u8)
            n187 = Add(x=w463, y=w459) -> (x+y=w464:u8)
            n188 = Select(t=DisplacementSampleSensorLoopStates."ReadErrorCR" ("State"), s=w461, f=DisplacementSampleSensorLoopStates."ResponseInvalidError" ("State")) -> (s? t:f=w467:T2)
            n189 = Bundle By Name(cluster=w469, "State"=w467, "ErrorNumber"=w464, "Timeout"=0) -> (w468:T1)
          }
        }
      }
      frame "ReadErrorCR" {
        n190 = xnode ("FIFO Method Node")("Timeout"=0) -> ("Element"=w470:u8, "Timed Out?"=w471:bool)  [unwired: 1 in, 1 out]
        n191 = case shown="False" w471 {
          tunnel: w474 -> [w476 w485]
          tunnel: [w475 w484] -> w473
          tunnel: w470 -> [_ w480]
          frame True {
            n192 = call "DisplacementCheckForTimeout.vi"("DisplacementSampleSensorLoopData in"=w476) -> ("DisplacementSampleSensorLoopData out"=w475:T1)  [unwired: 10 in]
          }
          frame False {
            # "\\r"
            n193 = Equal?(x=w480, y=u8 13) -> (x = y?=w479:bool)
            n194 = Select(t=DisplacementSampleSensorLoopStates."ParseErrorNumber" ("State"), s=w479, f=DisplacementSampleSensorLoopStates."ResponseInvalidError") -> (s? t:f=w478:T2)
            n195 = Bundle By Name(cluster=w485, "State"=w478, "Timeout"=0) -> (w484:T1)
          }
        }
      }
      frame "ParseErrorNumber" {
        n196 = case shown="255, Default" w486 {
          tunnel: [DisplacementSampleSensorLoopStates."ResponseInvalidError" ("State") DisplacementSampleSensorLoopStates."SensorIndicatesInvalidCommandError" ("State") DisplacementSampleSensorLoopStates."SensorIndicatesCommunicationTimeoutError" ("State") DisplacementSampleSensorLoopStates."SensorIndicatesDataLengthError" ("State") DisplacementSampleSensorLoopStates."SensorIndicatesNumberOfParametersError" ("State") DisplacementSampleSensorLoopStates."SensorIndicatesParameterError" ("State") DisplacementSampleSensorLoopStates."SensorIndicatesCommunicationError" ("State") DisplacementSampleSensorLoopStates."SensorIndicatesIDNumberError" ("State") DisplacementSampleSensorLoopStates."SensorIndicatesExpansionLineError" ("State") DisplacementSampleSensorLoopStates."SensorIndicatesWriteControlError" ("State")] -> w487
          frame 255, Default {
          }
          frame 0 {
          }
          frame 2 {
          }
          frame 20 {
          }
          frame 21 {
          }
          frame 22 {
          }
          frame 29 {
          }
          frame 65 {
          }
          frame 66 {
          }
          frame 67 {
          }
        }
        n197 = Bundle By Name(cluster=w489, "State"=w487) -> (w488:T1)
      }
      frame "ResponseUnknownError" {
        n198 = Bundle By Name(cluster=w503, "State"=DisplacementSampleSensorLoopStates."PrepareErrorCode", "ErrorSample.ErrorCode"=DisplacementErrorCodes."ResponseUnknownError" ("DisplacementErrorCodes")) -> (w502:T1)
      }
      frame "ResponseInvalidError" {
        n199 = Bundle By Name(cluster=w507, "State"=DisplacementSampleSensorLoopStates."PrepareErrorCode", "ErrorSample.ErrorCode"=DisplacementErrorCodes."ResponseInvalidError" ("DisplacementErrorCodes")) -> (w506:T1)
      }
      frame "ResponseTimeoutError" {
        n200 = Bundle By Name(cluster=w511, "State"=DisplacementSampleSensorLoopStates."PrepareErrorCode", "ErrorSample.ErrorCode"=DisplacementErrorCodes."ResponseTimeoutError" ("DisplacementErrorCodes")) -> (w510:T1)
      }
      frame "SensorIndicatesInvalidCommandError" {
        n201 = Bundle By Name(cluster=w515, "State"=DisplacementSampleSensorLoopStates."PrepareErrorCode", "ErrorSample.ErrorCode"=DisplacementErrorCodes."SensorIndicatesInvalidCommandError" ("DisplacementErrorCodes")) -> (w514:T1)
      }
      frame "SensorIndicatesCommunicationTimeoutError" {
        n202 = Bundle By Name(cluster=w519, "State"=DisplacementSampleSensorLoopStates."PrepareErrorCode", "ErrorSample.ErrorCode"=DisplacementErrorCodes."SensorIndicatesCommunicationTimeoutError" ("DisplacementErrorCodes")) -> (w518:T1)
      }
      frame "SensorIndicatesDataLengthError" {
        n203 = Bundle By Name(cluster=w523, "State"=DisplacementSampleSensorLoopStates."PrepareErrorCode", "ErrorSample.ErrorCode"=DisplacementErrorCodes."SensorIndicatesDataLengthError" ("DisplacementErrorCodes")) -> (w522:T1)
      }
      frame "SensorIndicatesNumberOfParametersError" {
        n204 = Bundle By Name(cluster=w527, "State"=DisplacementSampleSensorLoopStates."PrepareErrorCode", "ErrorSample.ErrorCode"=DisplacementErrorCodes."SensorIndicatesNumberOfParametersError" ("DisplacementErrorCodes")) -> (w526:T1)
      }
      frame "SensorIndicatesParameterError" {
        n205 = Bundle By Name(cluster=w531, "State"=DisplacementSampleSensorLoopStates."PrepareErrorCode", "ErrorSample.ErrorCode"=DisplacementErrorCodes."SensorIndicatesParameterError" ("DisplacementErrorCodes")) -> (w530:T1)
      }
      frame "SensorIndicatesCommunicationError" {
        n206 = Bundle By Name(cluster=w535, "State"=DisplacementSampleSensorLoopStates."PrepareErrorCode", "ErrorSample.ErrorCode"=DisplacementErrorCodes."SensorIndicatesCommunicationError" ("DisplacementErrorCodes")) -> (w534:T1)
      }
      frame "SensorIndicatesIDNumberError" {
        n207 = Bundle By Name(cluster=w539, "State"=DisplacementSampleSensorLoopStates."PrepareErrorCode", "ErrorSample.ErrorCode"=DisplacementErrorCodes."SensorIndicatesIDNumberError" ("DisplacementErrorCodes")) -> (w538:T1)
      }
      frame "SensorIndicatesExpansionLineError" {
        n208 = Bundle By Name(cluster=w543, "State"=DisplacementSampleSensorLoopStates."PrepareErrorCode", "ErrorSample.ErrorCode"=DisplacementErrorCodes."SensorIndicatesExpansionLineError" ("DisplacementErrorCodes")) -> (w542:T1)
      }
      frame "SensorIndicatesWriteControlError" {
        n209 = Bundle By Name(cluster=w547, "State"=DisplacementSampleSensorLoopStates."PrepareErrorCode", "ErrorSample.ErrorCode"=DisplacementErrorCodes."SensorIndicatesWriteControlError" ("DisplacementErrorCodes")) -> (w546:T1)
      }
      frame "PrepareErrorCode" {
        n210 = xnode ("Register Read")() -> ("Data"=w554:u64)  [unwired: 1 in, 1 out]
        n211 = xnode ("Register Read")() -> ("Data"=w550:u64)  [unwired: 1 in, 1 out]
        n212 = xnode ("Register Read")() -> ("Data"=w551:u64)  [unwired: 1 in, 1 out]
        n213 = xnode ("Register Read")() -> ("Data"=w549:u64)  [unwired: 1 in, 1 out]
        n214 = Increment(x=w554) -> (x+1=w552:u64)
        n215 = xnode ("Register Write")("Data"=w552) -> ()  [unwired: 1 in, 1 out]
        n216 = Bundle By Name(cluster=w557, "State"=DisplacementSampleSensorLoopStates."MoveErrorCode", "Sensor"=u8 1, "ErrorSample.RxFrames"=w552, "ErrorSample.TxBytes"=w551, "ErrorSample.RxBytes"=w550, "ErrorSample.TxFrames"=w549, "ErrorSample.Timestamp"=w548) -> (w556:T1)
      }
      frame "MoveErrorCode" {
        n217 = Unbundle By Name(w560) -> ("ErrorSample"=w558:T4)
        n218 = xnode ("FIFO Method Node")("Element"=w558, "Timeout"=0) -> ()  [unwired: 1 in, 2 out]
        n219 = Bundle By Name(cluster=w560, "State"=DisplacementSampleSensorLoopStates."WaitForTrigger", "Sensor"=u8 1) -> (w563:T1)
      }
    }
  }
  n220 = node-c288(w2) -> ()
